vi "String_Get Index.vi"(8 "error in (no error)":errorcluster, 9 "Default":string, 11 "Tag Name":string) -> (0 "error out":errorcluster, 3 "Index":i32)   [LabVIEW 2020, in "Current Value Table(Rebuild).lvlib"]
doc: "This VI retrieves the memory index of a single value as an I32. Since this value is an I32 and has no data associated with it, you must make sure that you use the index read and write for the appropriate type. This VI will check to make sure that the tag name specified matches with the data type specified."
uses:
  Current Value Table(Rebuild).lvlib
  FGVs/Tag Memory Methods.ctl
  String_Type To Enum.vi
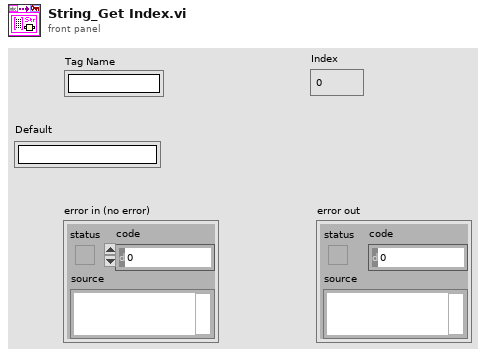
[diagram p1: front panel]
types:
  T1 = typedef "Current Value Table(Rebuild).lvlib/Tag Memory Methods.ctl" = enum16{"Clear", "Read Tag Index", "Read Tag Indices", "Generate Group", "Add Tag", "Overwrite Tag", "Read Description", "Get Stored Tags", "Write Description"}
  T2 = typedef "Current Value Table(Rebuild).lvlib/Data Types.ctl" = enum16{"Double", "Single", "I64", "I32", "I16", "I8", "U64", "U32", "U16", "U8", "String", "Boolean", "Array of U8", "Array of U16", "Array of U32", "Array of U64", "Array of I64", "Array of I32", "Array of I16", "Array of I8", "Array of Double", "Array of Single", "Array of Boolean", "Array of String"}
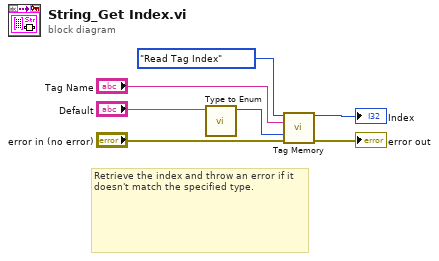
[diagram p0: block diagram]
diagram:
  # "Retrieve the index and throw an error if it doesn't match the specified type."
  n1 = call-poly "Type to Enum.vi"("Default"="Default") -> ("Data Type Enum"=w7:T2)  [unwired: 10 in]
  n2 = call "Tag Memory.vi"("Method"=Tag_Memory_Methods."Read Tag Index", "Tag"="Tag Name", "Expected Type"=w7, "error in (no error)"="error in (no error)") -> ("Index Out"=→"Index":i32, "error out"=→"error out":errorcluster)  [unwired: 6 in, 4 out]
